vi "Focus Standard Variation.vi"(8 "error in":errorcluster, 9 "Scan Increments":dbl=0.01 format="%#_13g", 10 "Component":T1, 11 "Gantry In":refnum<k24>) -> (0 "error out":errorcluster, 2 "max value":dbl, 3 "Gantry Out":refnum<k24>)   [LabVIEW 2021, in "Component Tray.lvclass"]
uses:
  Component/Component Tray.lvclass
  C:/Program Files (x86)/Aerotech/A3200/LabVIEW/2010/Bin/Aerotech.A3200.dll
  Program Files (x86)/Aerotech/A3200/LabVIEW/2010/Bin/Aerotech.A3200.dll
  Component/Find Component.ctl
  Controller/Camera/Machine Vision.ctl
  Controller/Motion/A3200/A3200.lvclass
  Controller/Camera/Camera.lvclass
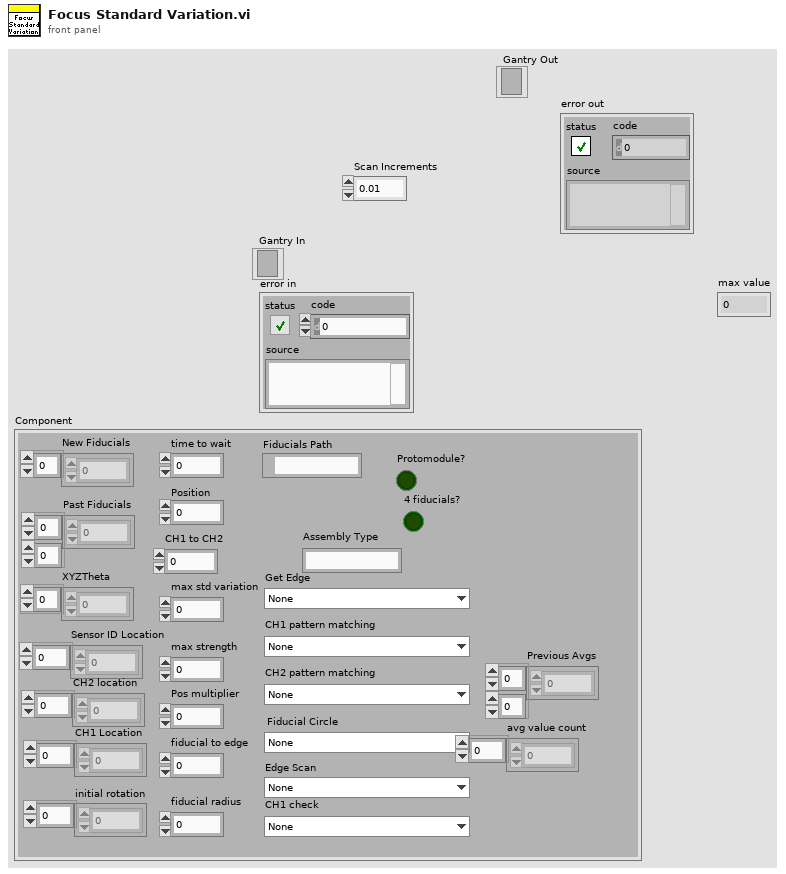
[diagram p1: front panel]
types:
  T1 = typedef "Component Tray.lvclass/Find Component.ctl" = cluster{"New Fiducials":dbl[], "Past Fiducials":dbl[][], "XYZTheta":dbl[], "Fiducials Path":path, "Position":i32, "CH1 Location":dbl[], "Sensor ID Location":dbl[], "initial rotation":dbl[], "CH2 location":dbl[], "max std variation":dbl, "max strength":dbl, "CH2 pattern matching":T2, "Fiducial Circle":T2, "Get Edge":T2, "Pos multiplier":dbl, "time to wait":u32, "fiducial to edge":dbl, "Protomodule?":bool, "Assembly Type":string, "CH1 to CH2":dbl, "Tray Number":string, "fiducial radius":dbl, "4 fiducials?":bool, "CH1 check":T2, "Edge Scan":T2, "CH1 pattern matching":T2, "Sensor Thickness":dbl, "Previous Avgs":dbl[][], "avg value count":dbl[]}
  T2 = typedef "Camera.lvclass/Machine Vision.ctl" = enum16{"None", "Assembly Tray Circle", "Assembly Tray Fiducial", "Partial Hexaboard", "sensor edge init", "HB edge init", "sensor edge pos1", "sensor edge pos2", "HB edge pos1", "HB edge pos2", "Sensor CH1-2", "HB CH1", "HB CH2", "V3 Sensor Circle", "Hexaboard Circle", "sensor CH1 check", "HB CH1 check ", "sensor ID"}
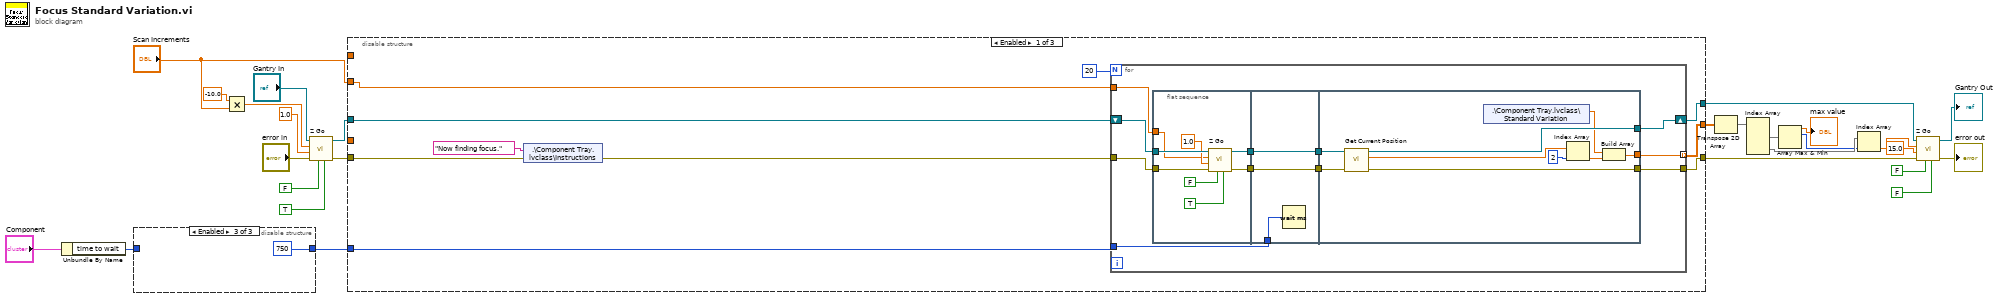
[diagram p0: block diagram]
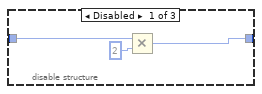
[diagram p2: hidden frame]
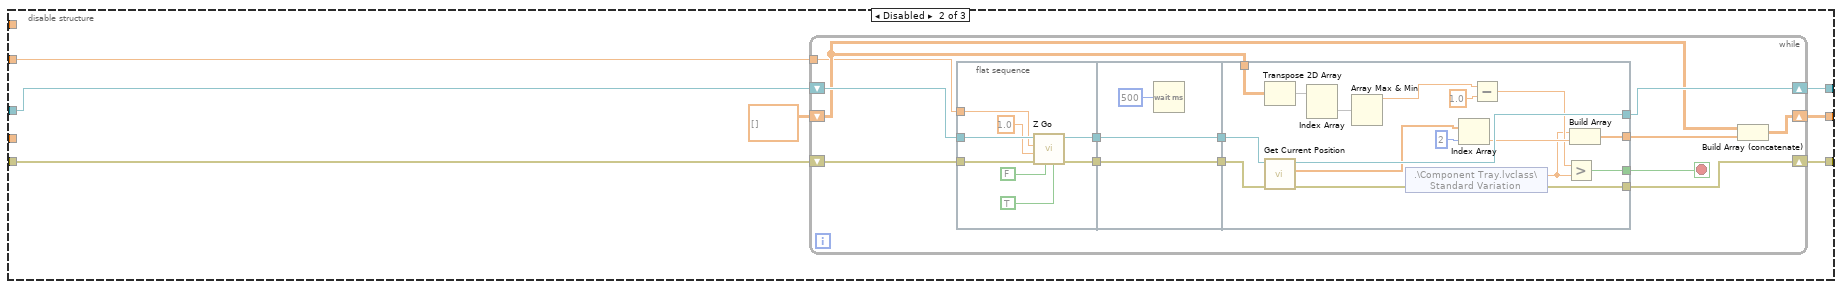
[diagram p4: hidden frame]
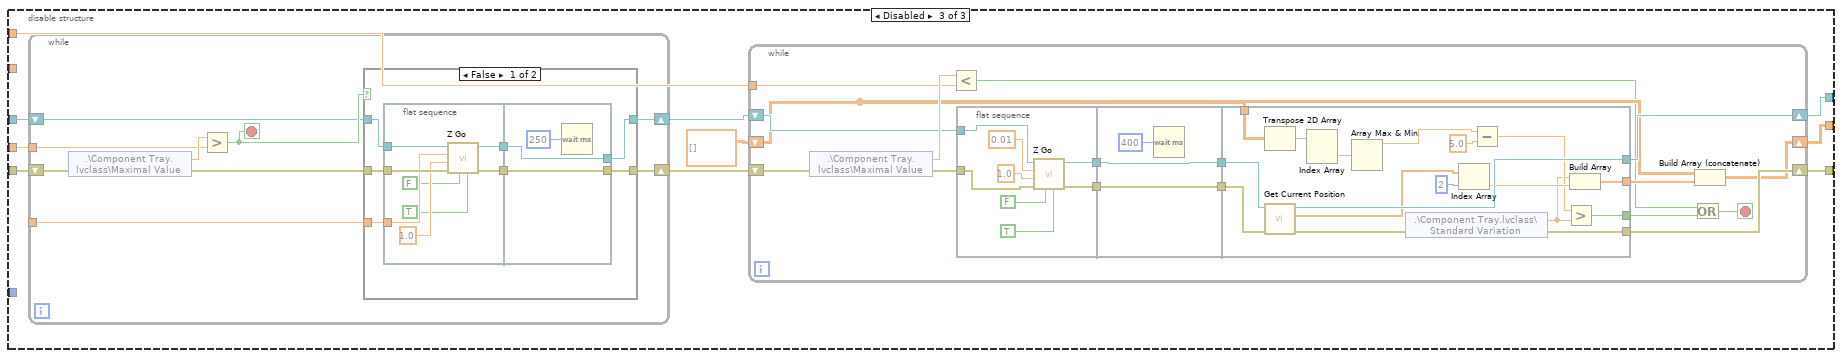
[diagram p5: hidden frame]
diagram:
  n1 = Unbundle By Name("Component") -> ("time to wait"=w2:u32)
  n2 = disable-structure shown="Enabled" {
    disable-tunnel: w2 -> [w30 w31 _]
    disable-tunnel: [w28 w31 u32 750] -> w1
    frame Disabled {
      n3 = Multiply(x=w30, y=u32 2) -> (x*y=w28:u32)
    }
    frame Disabled {
    }
    frame Enabled {
    }
  }
  n4 = Multiply(x=-10.0, y="Scan Increments") -> (x*y=w4:dbl)
  n5 = call "Z Go.vi"("Increment"=TRUE, "Return Immediately"=FALSE ("Increment"), "error in (no error)"="error in", "Speed In"=1.0 ("Speed"), "Position In"=w4, "Gantry In"="Gantry In") -> ("error out"=w9:errorcluster, "Gantry Out"=w10:refnum<k24>)  [unwired: 2 in, 2 out]
  n6 = disable-structure shown="Enabled" {
    disable-tunnel: [w42 w76 w125] -> w24
    disable-tunnel: [w41 w77 w126] -> w21
    disable-tunnel: [w40 w78 w128] -> w20
    disable-tunnel: w10 -> [w39 w80 w131]
    disable-tunnel: w9 -> [w36 w79 w130]
    disable-tunnel: _ -> [_ _ w123]
    disable-tunnel: _ -> [_ _ w122]
    disable-tunnel: "Scan Increments" -> [w38 w74 _]
    disable-tunnel: w1 -> [w33 _ _]
    frame Enabled {
      n7 = shared-variable ".\\Component Tray.lvclass\\Instructions"("Now finding focus." ("Instructions"), error in=w36) -> (error out=w35:errorcluster)
      n8 = for {
        N: 20 -> [_]
        tunnel: [w51] -> w42 mode=indexing
        tunnel: w35 -> [w50]
        tunnel: [w49] -> w40
        shift-right: [w52] -> w41
        shift-left: w39 -> [w53]
        tunnel: w38 -> [w44]
        tunnel: w33 -> [w43]
        n9 = flat-sequence {
          tunnel: w53 -> [w61]
          tunnel: [w60] -> w48
          tunnel: w50 -> [w59]
          tunnel: [w58] -> w46
          tunnel: w44 -> [w56]
          tunnel: w48 -> [w64]
          tunnel: [w64] -> w47
          tunnel: w46 -> [w63]
          tunnel: [w63] -> w45
          tunnel: w43 -> [w62]
          tunnel: w47 -> [w73]
          tunnel: [w72] -> w52
          tunnel: [w71] -> w51
          tunnel: w45 -> [w70]
          tunnel: [w69] -> w49
          frame #0 {
            n10 = call "Z Go.vi"("Increment"=TRUE, "Return Immediately"=FALSE ("Increment"), "error in (no error)"=w59, "Speed In"=1.0 ("Speed"), "Position In"=w56, "Gantry In"=w61) -> ("error out"=w58:errorcluster, "Gantry Out"=w60:refnum<k24>)  [unwired: 2 in, 2 out]
          }
          frame #1 {
            n11 = Wait (ms)(milliseconds to wait=w62) -> ()  [unwired: 1 out]
          }
          frame #2 {
            n12 = call "Get Current Position.vi"("error in (no error)"=w70, "Gantry In"=w73) -> ("error out"=w69:errorcluster, "XYZTheta Out"=w68:dbl[], "Gantry Out"=w72:refnum<k24>)  [unwired: 7 in]
            n13 = shared-variable ".\\Component Tray.lvclass\\Standard Variation"() -> (w65:sgl)  [unwired: 1 in, 1 out]
            n14 = Index Array(array=w68, index=2) -> (element=w66:dbl)
            n15 = Build Array(w65, w66) -> (w71:dbl[])
          }
        }
      }
    }
    frame Disabled {
      n16 = while {
        shift-right: [w85] -> w76
        shift-left: dbl[][] [] -> [w84]
        shift-right: [w91] -> w77
        shift-left: w80 -> [w92]
        shift-right: [w93] -> w78
        shift-left: w79 -> [w82]
        tunnel: w74 -> [w81]
        stop <- w83 stop-if-true
        n17 = flat-sequence {
          tunnel: w92 -> [w101]
          tunnel: [w100] -> w90
          tunnel: w82 -> [w99]
          tunnel: [w98] -> w89
          tunnel: w81 -> [w94]
          tunnel: w90 -> [w104]
          tunnel: [w104] -> w88
          tunnel: w89 -> [w103]
          tunnel: [w103] -> w87
          tunnel: w88 -> [w121]
          tunnel: [w120] -> w91
          tunnel: [w119] -> w86
          tunnel: w87 -> [w115]
          tunnel: [w113] -> w93
          tunnel: w84 -> [w112]
          tunnel: [w105] -> w83
          frame #0 {
            n18 = call "Z Go.vi"("Increment"=TRUE, "Return Immediately"=FALSE ("Increment"), "error in (no error)"=w99, "Speed In"=1.0 ("Speed"), "Position In"=w94, "Gantry In"=w101) -> ("error out"=w98:errorcluster, "Gantry Out"=w100:refnum<k24>)  [unwired: 2 in, 2 out]
          }
          frame #1 {
            n19 = Wait (ms)(milliseconds to wait=u32 500) -> ()  [unwired: 1 out]
          }
          frame #2 {
            n20 = Transpose 2D Array(2D array=w112) -> (transposed array=w111:dbl[][])
            n21 = call "Get Current Position.vi"("error in (no error)"=w115, "Gantry In"=w121) -> ("error out"=w114:errorcluster, "XYZTheta Out"=w118:dbl[], "Gantry Out"=w120:refnum<k24>)  [unwired: 7 in]
            n22 = Index Array(array=w111) -> (element=w110:dbl[])  [unwired: 2 in]
            n23 = Array Max & Min(array=w110) -> (max value=w109:dbl)  [unwired: 3 out]
            n24 = shared-variable ".\\Component Tray.lvclass\\Standard Variation"(error in=w114) -> (w106:sgl, error out=w113:errorcluster)
            n25 = Index Array(array=w118, index=2) -> (element=w116:dbl)
            n26 = Subtract(x=w109, y=1.0) -> (x-y=w107:dbl)
            n27 = Greater?(x=w107, y=w106) -> (0:w105:bool)
            n28 = Build Array(w106, w116) -> (w119:dbl[])
          }
        }
        n29 = Build Array (concatenate)(w84, w86) -> (w85:dbl[][])
      }
    }
    frame Disabled {
      n30 = while {
        shift-right: [w182] -> w127
        shift-left: w131 -> [w183]
        shift-right: [w181] -> w129
        shift-left: w130 -> [w179]
        tunnel: _ -> [w180]
        tunnel: w123 -> [w177]
        stop <- w184 stop-if-true
        n31 = shared-variable ".\\Component Tray.lvclass\\Maximal Value"(error in=w179) -> (w185:sgl, error out=w178:errorcluster)
        n32 = Greater?(x=w185, y=w177) -> (0:w184:bool)
        n33 = case shown="False" w184 {
          tunnel: w183 -> [w190 w205]
          tunnel: [w187 w205] -> w182
          tunnel: [w186 w204] -> w181
          tunnel: w178 -> [w189 w204]
          tunnel: w180 -> [w188 _]
          frame False {
            n34 = flat-sequence {
              tunnel: w190 -> [w200]
              tunnel: [w199] -> w192
              tunnel: w189 -> [w198]
              tunnel: [w197] -> w191
              tunnel: w188 -> [w195]
              tunnel: w192 -> [w202]
              tunnel: w191 -> [w201]
              tunnel: [w202] -> w187
              tunnel: [w201] -> w186
              frame #0 {
                n35 = call "Z Go.vi"("Increment"=TRUE, "Return Immediately"=FALSE ("Increment"), "error in (no error)"=w198, "Speed In"=1.0 ("Speed"), "Position In"=w195, "Gantry In"=w200) -> ("error out"=w197:errorcluster, "Gantry Out"=w199:refnum<k24>)  [unwired: 2 in, 2 out]
              }
              frame #1 {
                n36 = Wait (ms)(milliseconds to wait=u32 250) -> ()  [unwired: 1 out]
              }
            }
          }
          frame True {
          }
        }
      }
      n37 = while {
        shift-right: [w137] -> w125
        shift-left: dbl[][] [] -> [w135]
        tunnel: w122 -> [w136]
        shift-right: [w145] -> w126
        shift-left: w127 -> [w146]
        shift-right: [w147] -> w128
        shift-left: w129 -> [w144]
        stop <- w133 stop-if-true
        n38 = shared-variable ".\\Component Tray.lvclass\\Maximal Value"(error in=w144) -> (w148:sgl, error out=w143:errorcluster)
        n39 = Less?(x=w148, y=w136) -> (x < y?=w134:bool)
        n40 = flat-sequence {
          tunnel: w146 -> [w156]
          tunnel: [w155] -> w142
          tunnel: w143 -> [w154]
          tunnel: [w153] -> w141
          tunnel: w142 -> [w159]
          tunnel: [w159] -> w140
          tunnel: w141 -> [w158]
          tunnel: [w158] -> w139
          tunnel: w140 -> [w176]
          tunnel: [w175] -> w145
          tunnel: [w174] -> w138
          tunnel: w139 -> [w170]
          tunnel: [w168] -> w147
          tunnel: w135 -> [w167]
          tunnel: [w160] -> w132
          frame #0 {
            n41 = call "Z Go.vi"("Increment"=TRUE, "Return Immediately"=FALSE ("Increment"), "error in (no error)"=w154, "Speed In"=1.0 ("Speed"), "Position In"=0.01, "Gantry In"=w156) -> ("error out"=w153:errorcluster, "Gantry Out"=w155:refnum<k24>)  [unwired: 2 in, 2 out]
          }
          frame #1 {
            n42 = Wait (ms)(milliseconds to wait=u32 400) -> ()  [unwired: 1 out]
          }
          frame #2 {
            n43 = Transpose 2D Array(2D array=w167) -> (transposed array=w166:dbl[][])
            n44 = call "Get Current Position.vi"("error in (no error)"=w170, "Gantry In"=w176) -> ("error out"=w169:errorcluster, "XYZTheta Out"=w173:dbl[], "Gantry Out"=w175:refnum<k24>)  [unwired: 7 in]
            n45 = Index Array(array=w166) -> (element=w165:dbl[])  [unwired: 2 in]
            n46 = Array Max & Min(array=w165) -> (max value=w164:dbl)  [unwired: 3 out]
            n47 = shared-variable ".\\Component Tray.lvclass\\Standard Variation"(error in=w169) -> (w161:sgl, error out=w168:errorcluster)
            n48 = Index Array(array=w173, index=2) -> (element=w171:dbl)
            n49 = Subtract(x=w164, y=5.0) -> (x-y=w162:dbl)
            n50 = Greater?(x=w162, y=w161) -> (0:w160:bool)
            n51 = Build Array(w161, w171) -> (w174:dbl[])
          }
        }
        n52 = Or(x=w134, y=w132) -> (x .or. y?=w133:bool)
        n53 = Build Array (concatenate)(w135, w138) -> (w137:dbl[][])
      }
    }
  }
  n54 = Transpose 2D Array(2D array=w24) -> (transposed array=w14:dbl[][])
  n55 = Index Array(array=w14) -> (element #1=w11:dbl[], element #2=w13:dbl[])  [unwired: 4 in]
  n56 = Array Max & Min(array=w11) -> (max value=→"max value":dbl, max index (indices)=w12:i32)  [unwired: 2 out]
  n57 = Index Array(array=w13, index=w12) -> (element=w23:dbl)
  n58 = call "Z Go.vi"("Increment"=FALSE, "Return Immediately"=FALSE ("Increment"), "error in (no error)"=w20, "Speed In"=15.0 ("Speed"), "Position In"=w23, "Gantry In"=w21) -> ("error out"=→"error out":errorcluster, "Gantry Out"=→"Gantry Out":refnum<k24>)  [unwired: 2 in, 2 out]
